vi "Robot Global Data.vi"() -> ()   [LabVIEW 2019]
doc: "This global VI can contain as many global variables as you need. Place a control on the panel, give it a good name. To read or write to it from a VI, drag the icon to the diagram of that VI. You can also drag from the project. Click on the node to change which global you access. You shouldn't have multiple locations writing to a global or it will cause a race-condition."
uses:
  <vilib>/Rock Robotics/WPI/Camera/WPI_CameraImageSize.ctl
  <vilib>/Rock Robotics/WPI/DriverStation/WPI_DriverStationRobotMode2.ctl
panel:
  out "RPM Gauge":dbl
  out "Gyro Offset":dbl
  out "X PID":dbl
  out "X Offset":dbl
  out "X Wanted Auto":dbl
  out "Turret Gyro":dbl
  out "Auto Intake":bool
  out "Auto Shoot":bool
  out "Int Pos":bool
  out "y Int":dbl
  out "x Int":dbl
  out "Range":dbl
  out "Wanted Turret Angle":dbl
  out "Shooter Speed":dbl
  out "Feeder Speed":dbl
  out "Conveyer Speed":dbl
  out "Intake Speed":dbl
  out "X Absolute Angle":dbl
  out "X Relative Angle":dbl
  out "Wheel Drive Encoders":cluster{"Rates":dbl[], "Distances":dbl[]}={"Rates"=[0.0, 0.0, -0.0, -0.0], "Distances"=[195.26625, 229.86928250000003, -80.247456, 179.07341]}
  out "y Vel":dbl
  out "x Vel":dbl
  out "Heading":dbl
  out "Auto X":dbl
  out "y Pos":dbl
  out "x Pos":dbl
  out "Auto Y":dbl
  out "Reset All":bool
  out "Auto Controls":bool
  out "Rot Pt Y":dbl
  out "Rot Pt X":dbl
  out "Gyro Angle":dbl(knob) scale=0.0..360.0
  out "Reset Gyro":bool
  out "Robot Centric":bool
  out "z":dbl
  out "y":dbl
  out "x":dbl
  in  "Robot Mode":T1
  in  "image size":T2=enum."320x240"
  in  "Enable Vision":bool
  # "Drive Control\nValues"
  # "Robot Rotation\nPoint"
  # "Vision Data"
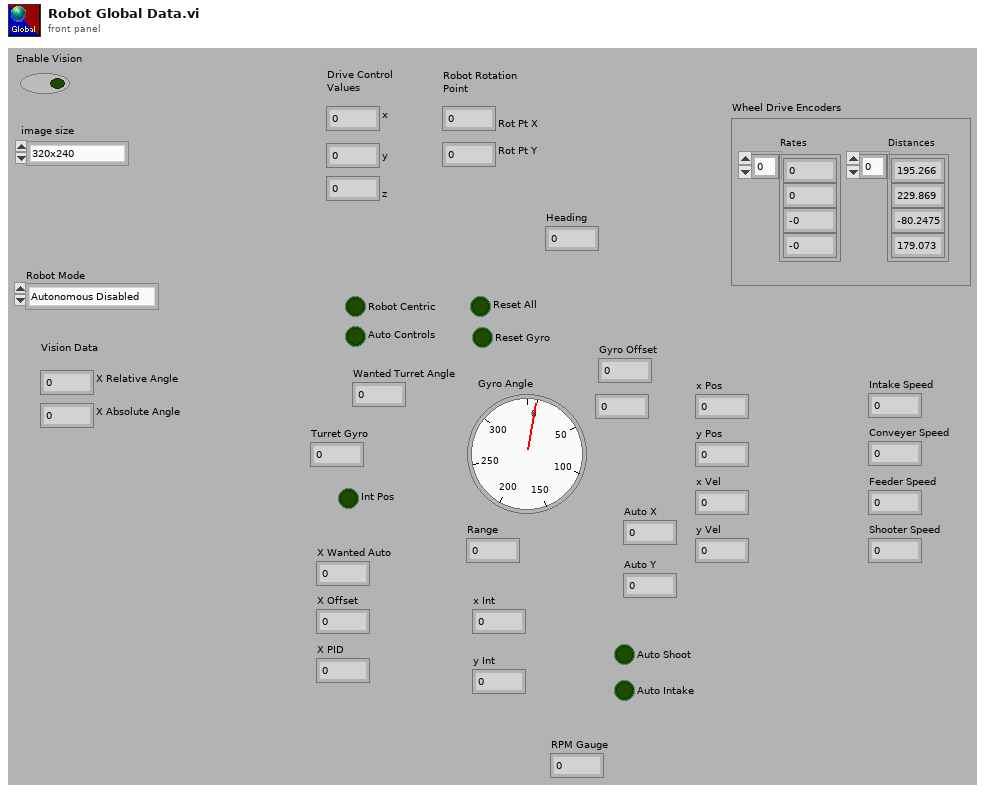
[diagram p1: front panel]
types:
  T1 = typedef "WPI_DriverStationRobotMode2.ctl" = enum16{"Autonomous Disabled", "Autonomous Enabled", "Teleop Disabled", "Teleop Enabled", "Disconnected", "Finish", "Test Disabled", "Test Enabled", "Emergency Stopped"}
  T2 = typedef "WPI_CameraImageSize.ctl" = enum16{"640x480", "320x240", "160x120", "Custom"}
diagram:
